vi "Acquire_Data.vi"() -> (4 "Binary output":i16[][](array[numeric])=[[-1019, -892, -715, -592, -607, -745, -922, -1028, -992, -843], [-1000, -852, -680, -586, -636, -796, -963, -1039, -967, -802], [187, 183, 188, 180, 191, 182, 193, 184, 188, 185]], 10 "Block Timings":T1={"Started"=0.0, "Ended"=0.0, "Analogue Frequency Hz"=1000.0} {"Analogue Frequency Hz" format="%.2f"}, 15 "error out":errorcluster)   [LabVIEW 2010]
doc: "Paul- there seems to be a bit of a problem if you use the channels out of order; you have to use them starting from ch 0 and consecutive nos. above that. I'm not sure why; note- I return my channels in the order the user used them, not lowest first; does this make a difference. If it needs changing, do it in the ADC kernel; thats where I want to keep all the compatibility re-mappings.\nActually, the problem may be if you don't use channel 0?....."
uses:
  Controls/Block_start_and_end.ctl
  ADAM Client/Sub VIs/ADAM Controls/Traverse_Level_State.ctl
  Globals/Meas_global.vi
  Globals/Dynamic_call_global.ph.vi
panel:
  in  "No of Analogue Samples":i32=128 min=0 step=1
  in  "Analogue Sampling rate":dbl=100.0 format="%.2f"
  out "size(s)":i32[](array[numeric])
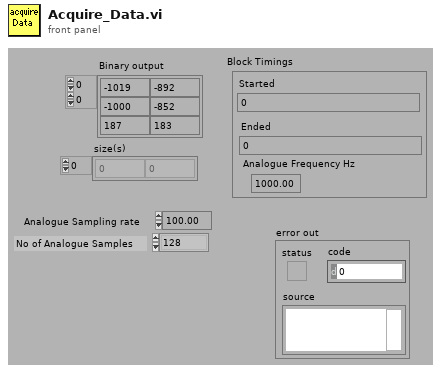
[diagram p1: front panel]
types:
  T1 = typedef "Block_start_and_end.ctl" = cluster{"Started":dbl, "Ended":dbl, "Analogue Frequency Hz":dbl}
  T2 = typedef "Ch_and_Spans.ctl" = cluster{"high limit (10V)":sgl, "low limit (-10V)":sgl, "Ch No":i16, "Var name":string, "Use Latest Calib":bool}
  T3 = typedef "Board_Types.ctl" = enum16{"Simulate", "NB-MIO-16H", "PCI-MIO-16E", "6000E Series", "USB-92xx", "ADC488", "Lab-NB", "NB-DIO-24", "NI-DAQmx", "Local ADAM", "Server Channels"}
  T4 = typedef "Traverse_Level_State.ctl" = enum16{"Running", "Complete"}
  T5 = typedef "Trigger_Mode.ctl" = enum16{"Free Running", "Start on Trigger", "Trigger Every Block", "Trigger Every Sample"}
  T6 = cluster{"channel":string, "upper input limits":sgl, "lower input limits":sgl, "range":sgl, "polarity":u16, "gain":sgl, "coupling":u16, "input mode":u16, "scale multiplier":dbl, "scale offset":dbl}[]
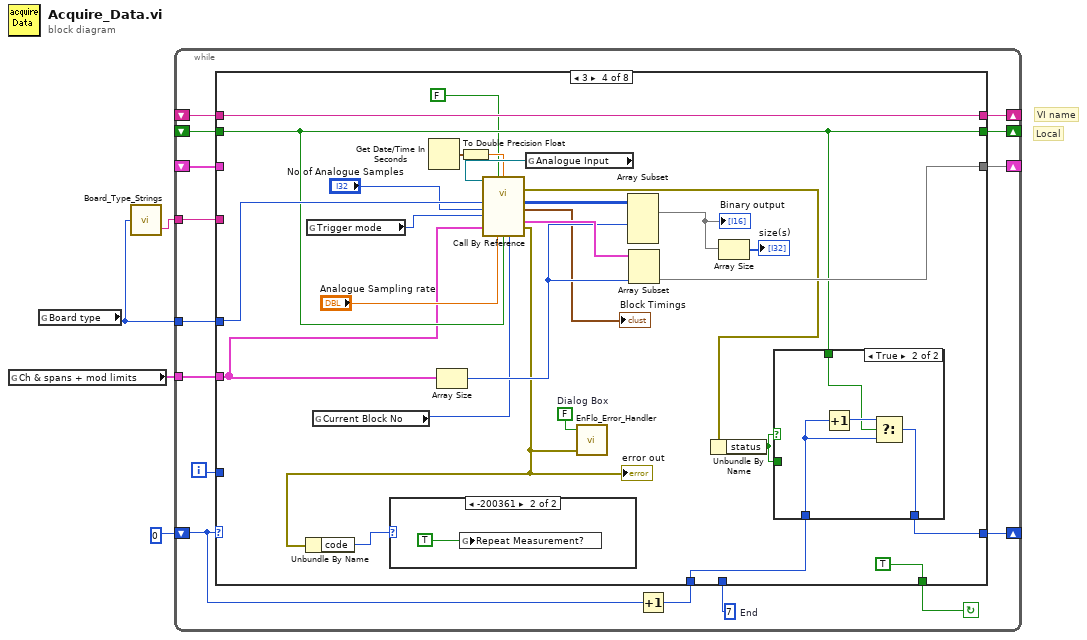
[diagram p0: block diagram]
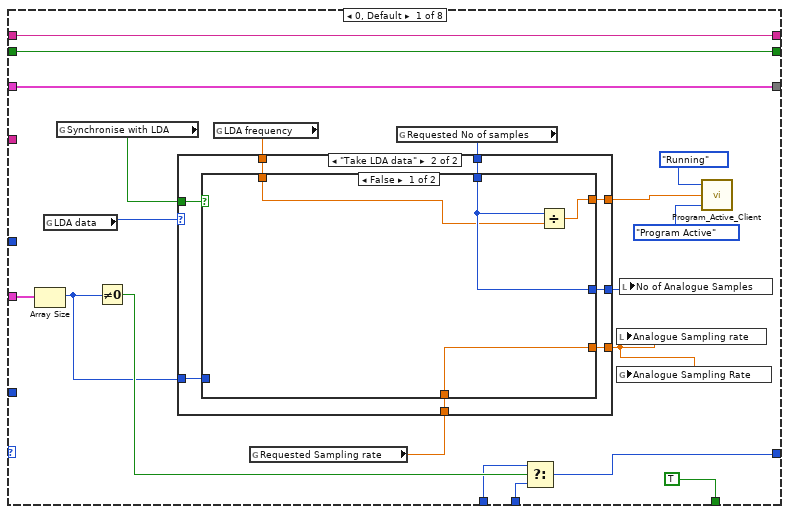
[diagram p2: hidden frame]
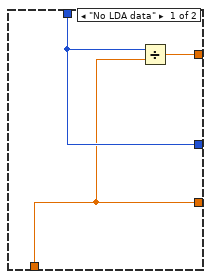
[diagram p3: hidden frame]
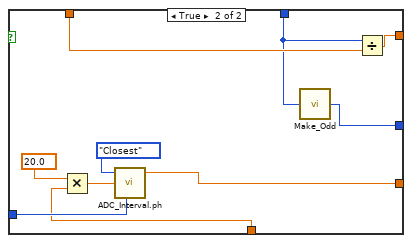
[diagram p4: hidden frame]
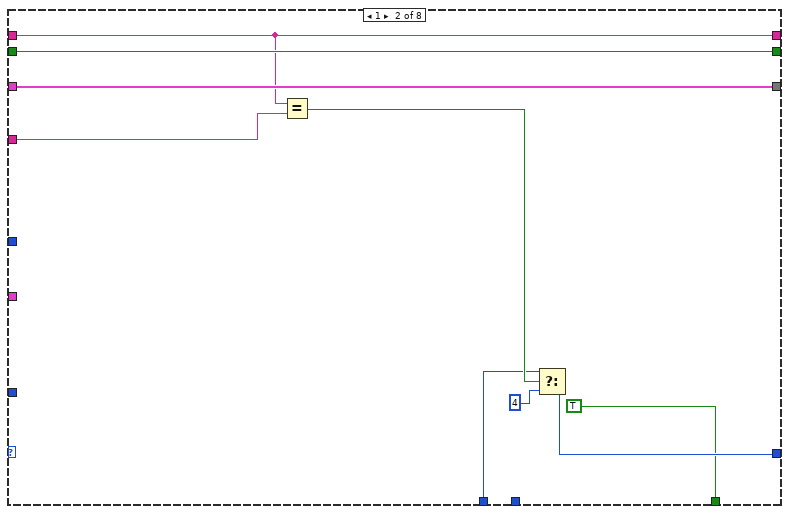
[diagram p5: hidden frame]
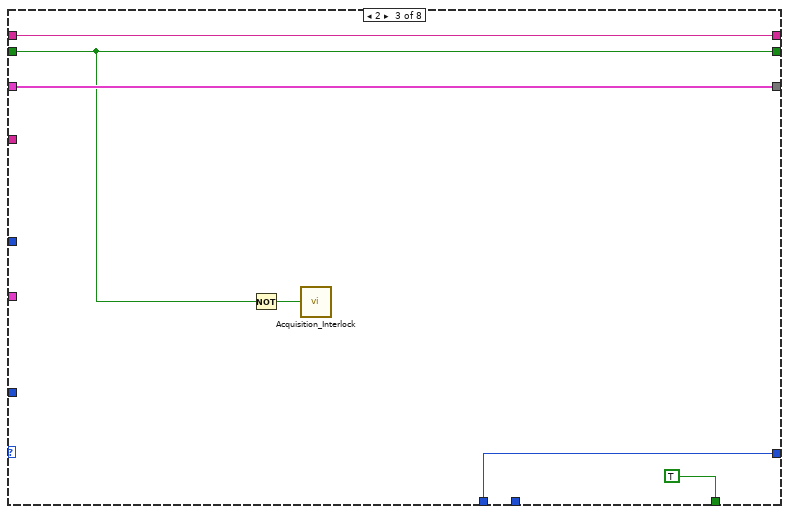
[diagram p6: hidden frame]
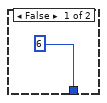
[diagram p8: hidden frame]
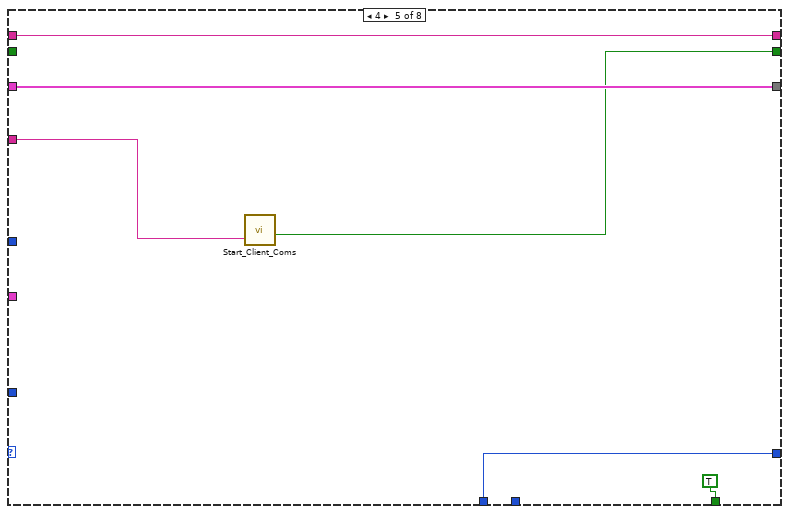
[diagram p9: hidden frame]
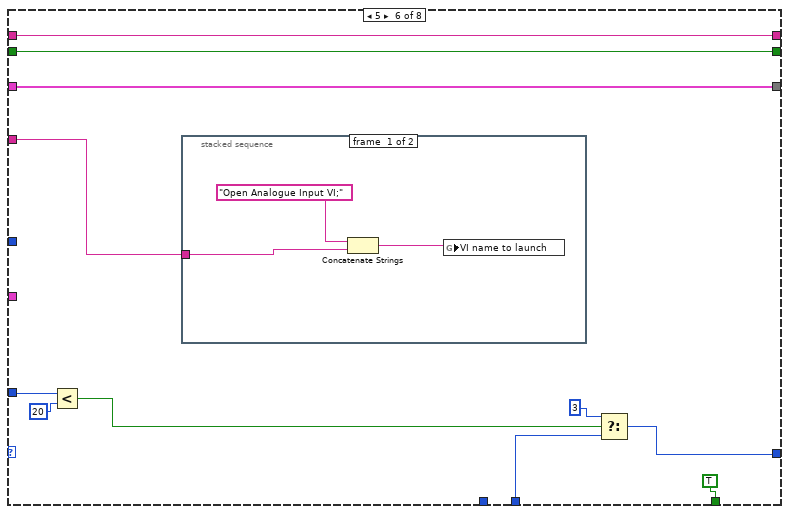
[diagram p10: hidden frame]
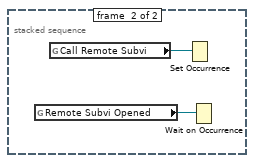
[diagram p11: hidden frame]
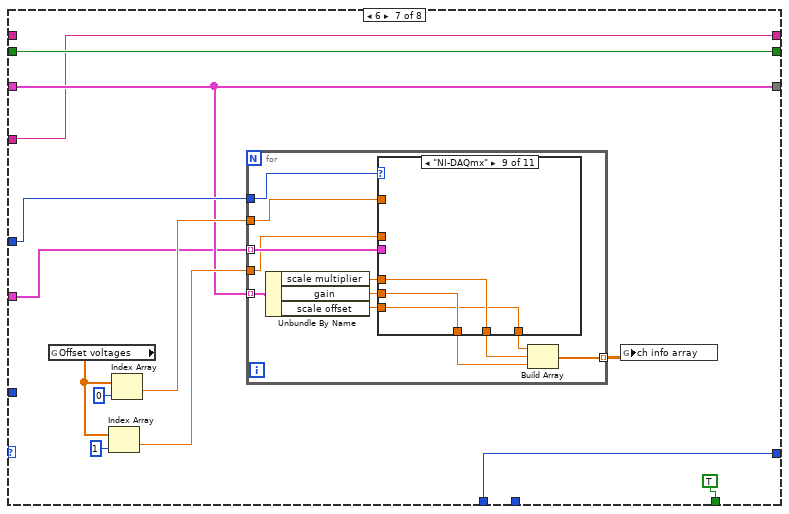
[diagram p12: hidden frame]
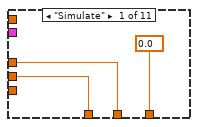
[diagram p13: hidden frame]
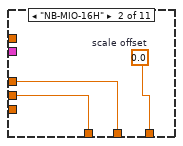
[diagram p14: hidden frame]
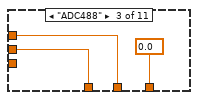
[diagram p15: hidden frame]
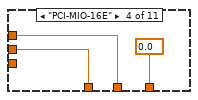
[diagram p16: hidden frame]
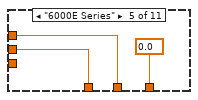
[diagram p17: hidden frame]
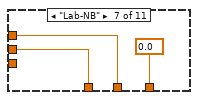
[diagram p19: hidden frame]
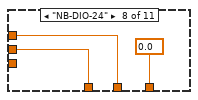
[diagram p20: hidden frame]
diagram:
  # "VI name"
  # "Local"
  n1 = global read "Meas_global.vi" "Ch & spans + mod limits"() -> (w3:T2[])
  n2 = global read "Meas_global.vi" "Board type"() -> (w2:T3)
  n3 = call "Board_Type_Strings.vi"("Board type"=w2) -> ("Acquisition VI Name"=w1:string)  [unwired: 1 out]
  n4 = while {
    tunnel: w1 -> [w5]
    shift-left: _ -> [w6]
    shift-right: [w7] -> _
    shift-left: _ -> [w9]
    shift-right: [w10] -> _
    shift-left: _ -> [w11]
    shift-right: [w12] -> _
    tunnel: w2 -> [w13]
    tunnel: w3 -> [w15]
    shift-left: 0 -> [w19]
    shift-right: [w16] -> _
    i -> [w8]
    stop <- w18 continue-if-true
    w14 = 7  # End
    n5 = Increment(x=w19) -> (x+1=w17:i32)
    n6 = case shown="3" w19 {
      tunnel: [TRUE TRUE TRUE TRUE TRUE TRUE TRUE FALSE] -> w18
      tunnel: w17 -> [w35 w68 w76 w87 w117 _ w146 w196]
      tunnel: [w29 w71 w76 w97 w117 w121 w146 w196] -> w16
      tunnel: w15 -> [w38 _ _ w86 _ _ w137 _]
      tunnel: w14 -> [w36 _ _ _ _ w122 _ _]
      tunnel: w13 -> [_ _ _ w105 _ _ w142 _]
      tunnel: [w34 w73 w75 w93 w115 w129 w147 w197] -> w12
      tunnel: w11 -> [w34 w73 w75 w93 _ w129 w147 w197]
      tunnel: [w33 w66 w79 w106 w114 w120 w135 w194] -> w10
      tunnel: w9 -> [w33 w66 w79 w106 w114 w120 _ w194]
      tunnel: w8 -> [_ _ _ _ _ w125 _ _]
      tunnel: [w32 w69 w77 w99 w118 w128 w138 w193] -> w7
      tunnel: w6 -> [w32 w69 w77 _ w118 w128 w138 w193]
      tunnel: w5 -> [_ w65 _ _ w113 w119 w135 _]
      frame 0, Default {
        n7 = Array Size(array=w38) -> (size(s)=w25:i32)
        n8 = global read "Meas_global.vi" "LDA data"() -> (w31:enum16{"No LDA data", "Take LDA data"})
        n9 = global read "Meas_global.vi" "Synchronise with LDA"() -> (w30:bool)
        n10 = Not Equal To 0?(x=w25) -> (x != 0?=w37:bool)
        n11 = global read "Meas_global.vi" "LDA frequency"() -> (w21:dbl)
        n12 = global read "Meas_global.vi" "Requested Sampling rate"() -> (w26:dbl)
        n13 = global read "Meas_global.vi" "Requested No of samples"() -> (w27:i32)
        n14 = case shown="\"Take LDA data\"" w31 {
          tunnel: w30 -> [_ w50]
          tunnel: [w41 w49] -> w20
          tunnel: [w42 w48] -> w28
          tunnel: w27 -> [w42 w47]
          tunnel: w26 -> [w41 w46]
          tunnel: w25 -> [_ w45]
          tunnel: [w40 w43] -> w22
          tunnel: w21 -> [_ w44]
          frame "No LDA data" {
            n15 = Divide(x=w42, y=w41) -> (x/y=w40:dbl)
          }
          frame "Take LDA data" {
            n16 = case shown="False" w50 {
              tunnel: [w54 w60] -> w49
              tunnel: [w52 w57] -> w48
              tunnel: w47 -> [w52 w56]
              tunnel: w46 -> [w54 w55]
              tunnel: w45 -> [_ w62]
              tunnel: w44 -> [w51 w58]
              tunnel: [w53 w59] -> w43
              frame False {
                n17 = Divide(x=w52, y=w51) -> (x/y=w53:dbl)
              }
              frame True {
                n18 = Multiply(x=20.0 ("y"), y=w55) -> (x*y=w64:dbl)
                n19 = call "ADC_Interval.ph.vi"("Frequency selection"=enum16{"Closest", "Next highest"}."Closest", "Sampling rate (Hz)"=w64, "number of channels"=w62) -> ("Actual Sampling Rate (Hz)"=w60:dbl)  [unwired: 1 in, 5 out]
                n20 = call "Make_Odd.vi"("No of samples"=w56) -> ("Odd No of Samples"=w57:i32)
                n21 = Divide(x=w56, y=w58) -> (x/y=w59:dbl)
              }
            }
          }
        }
        n22 = Select(t=w35, s=w37, f=w36) -> (s? t:f=w29:i32)
        n23 = local write "Analogue Sampling rate"(w20) -> ()
        n24 = global write "Meas_global.vi" "Analogue Sampling Rate"(w20) -> ()
        n25 = local write "No of Analogue Samples"(w28) -> ()
        n26 = call "Program_Active_Client.vi"("Mode"=enum16{"Program Active", "Traverse Level State"}."Program Active", "Time till next contact (Sec)"=w22, "Traverse level State"=Traverse_Level_State."Running") -> ()  [unwired: 3 out]
      }
      frame 1 {
        n27 = Equal?(x=w66, y=w65) -> (x = y?=w72:bool)
        n28 = Select(t=w68, s=w72, f=4) -> (s? t:f=w71:i32)
      }
      frame 2 {
        n29 = Not(x=w75) -> (.not. x?=w74:bool)
        n30 = call "Acquisition_Interlock.vi"("Local Control"=w74) -> ()
      }
      frame 3 {
        w92 = FALSE  # Dialog Box
        n31 = global read "Meas_global.vi" "Trigger mode"() -> (w84:T5)
        n32 = global read "Meas_global.vi" "Current Block No"() -> (w94:i32)
        n33 = Get Date/Time In Seconds() -> (seconds since 1Jan1904=w83:timestamp)
        n34 = Array Size(array=w86) -> (size(s)=w95:i32)
        n35 = To Double Precision Float(number=w83) -> (double precision float=w91:dbl)
        n36 = global read "Dynamic_call_global.ph.vi" "Analogue Input"() -> (w96:refnum<vi>)
        n37 = call-by-ref "?"(reference=w96, "Board type"=w105, "interval scanning"=FALSE, "Client Time"=w91, "No of samples+extra"="No of Analogue Samples", "Trigger mode"=w84, "Ch & spans"=w86, "Actual Sampling rate (Hz)"="Analogue Sampling rate", "Local Client?"=w93, "Current Block No"=w94) -> (error out=w98:errorcluster, "I16 data"=w103:i16[][], "Block Timings"=→"Block Timings":T1, "group channel settings"=w102:T6, "error out"=w82:errorcluster)  [unwired: 4 in, 1 out]
        "error out" <- w82
        n38 = Unbundle By Name(w82) -> ("code"=w81:i32)
        n39 = case shown="-200361" w81 {
          frame 0, Default {
          }
          frame -200361 {
            n40 = global write "Meas_global.vi" "Repeat Measurement?"(TRUE) -> ()
          }
        }
        n41 = call "EnFlo_Error_Handler.vi"("error in (no error)"=w82, "Dialog Box (T)"=w92) -> ()  [unwired: 1 in, 3 out]
        n42 = Array Subset(array=w103, length (row)=w95) -> (w100:i16[][])  [unwired: 3 in]
        "Binary output" <- w100
        n43 = Array Subset(array=w102, length=w95) -> (w99:T6)  [unwired: 1 in]
        n44 = Unbundle By Name(w98) -> ("status"=w90:bool)
        n45 = Array Size(array=w100) -> (size(s)=→"size(s)":i32[])
        n46 = case shown="True" w90 {
          tunnel: [6 ("f") w109] -> w97
          tunnel: w87 -> [_ w111]
          tunnel: w93 -> [_ w110]
          tunnel: w90 -> [_ _]
          frame False {
          }
          frame True {
            n47 = Increment(x=w111) -> (x+1=w112:i32)
            n48 = Select(t=w112, s=w110, f=w111) -> (s? t:f=w109:i32)
          }
        }
      }
      frame 4 {
        n49 = call "Start_Client_Coms.vi"("VI name to run on server"=w113) -> ("Local Call"=w115:bool)  [unwired: 1 in, 3 out]
      }
      frame 5 {
        n50 = Less?(x=w125, y=20) -> (x < y?=w124:bool)
        n51 = stacked-sequence {
          tunnel: w119 -> [w131 _]
          frame #0 {
            n52 = Concatenate Strings("Open Analogue Input VI;", w131) -> (w130:string)
            n53 = global write "Dynamic_call_global.ph.vi" "VI name to launch"(w130) -> ()
          }
          frame #1 {
            n54 = global read "Dynamic_call_global.ph.vi" "Remote Subvi Opened"() -> (w133:refnum<k4>)
            n55 = global read "Dynamic_call_global.ph.vi" "Call Remote Subvi"() -> (w134:refnum<k4>)
            n56 = Set Occurrence(w134) -> ()
            n57 = Wait on Occurrence(2:w133) -> ()  [unwired: 3 out]
          }
        }
        n58 = Select(t=3 ("f"), s=w124, f=w122) -> (s? t:f=w121:i32)
      }
      frame 6 {
        n59 = global read "Meas_global.vi" "Offset voltages"() -> (w141:dbl[])
        n60 = Index Array(array=w141, index=1) -> (element=w139:dbl)
        n61 = Index Array(array=w141, index=0) -> (element=w140:dbl)
        n62 = for {
          tunnel: w137 -> [w159] mode=indexing
          tunnel: w139 -> [w158]
          tunnel: w140 -> [w157]
          tunnel: [w155] -> w136 mode=indexing
          tunnel: w142 -> [w154]
          tunnel: w138 -> [w153] mode=indexing
          n63 = Unbundle By Name(w153) -> ("scale multiplier"=w151:dbl, "gain"=w149:sgl, "scale offset"=w148:dbl)
          n64 = case shown="\"NI-DAQmx\"" w154 {
            tunnel: w159 -> [_ _ _ _ _ _ _ _ _ _ _]
            tunnel: w158 -> [_ _ _ _ _ _ _ _ _ _ _]
            tunnel: w157 -> [_ _ _ _ _ _ _ _ _ _ _]
            tunnel: [0.0 w163 0.0 0.0 0.0 w175 0.0 0.0 w184 w187 w190] -> w156
            tunnel: [w161 w165 w167 w170 w173 w177 w179 w182 w186 w189 w192] -> w152
            tunnel: w151 -> [w161 w165 w167 w170 w173 w177 w179 w182 w186 w189 w192]
            tunnel: [w160 w164 w166 w169 w172 w176 w178 w181 w185 w188 w191] -> w150
            tunnel: w149 -> [w160 w164 w166 w169 w172 w176 w178 w181 w185 w188 w191]
            tunnel: w148 -> [_ _ _ _ _ w175 _ _ w184 w187 w190]
            frame "Simulate" {
            }
            frame "NB-MIO-16H" {
              w163 = 0.0  # scale offset
            }
            frame "ADC488" {
            }
            frame "PCI-MIO-16E" {
            }
            frame "6000E Series" {
            }
            frame "USB-92xx" {
            }
            frame "Lab-NB" {
            }
            frame "NB-DIO-24" {
            }
            frame "NI-DAQmx" {
            }
            frame "Local ADAM" {
            }
            frame "Server Channels" {
            }
          }
          n65 = Build Array(w156, w152, w150) -> (w155:dbl[])
        }
        n66 = global write "Meas_global.vi" "ch info array"(w136) -> ()
      }
      frame 7 {
      }
    }
  }
